vi "RVHR - New Distance.vi"(5 "Command":enum16{"Next", "Previous"}(ring), 6 "Local Data in":T3, 7 "UI Refs":T2, 8 "error in (no error)":errorcluster, 11 "Supervisory Config Cluster In":T1) -> (0 "error out":errorcluster, 3 "New Distance":dbl, 4 "Local Data out":T3)   [LabVIEW 2024]
uses:
  Controls/RVHR - Local Data.ctl
  Controls/Test Cluster.ctl
  Controls/Excluded Information.ctl
  Controls/Language.ctl
  Controls/Device_Type.ctl
  <vilib>/Utility/miscctls.llb/LVRectTypeDef.ctl
  <vilib>/Utility/miscctls.llb/LVBoundsTypeDef.ctl
  Controls/RVHR - UI Refs.ctl
  Controls/RVHR - Reporting Settings.ctl
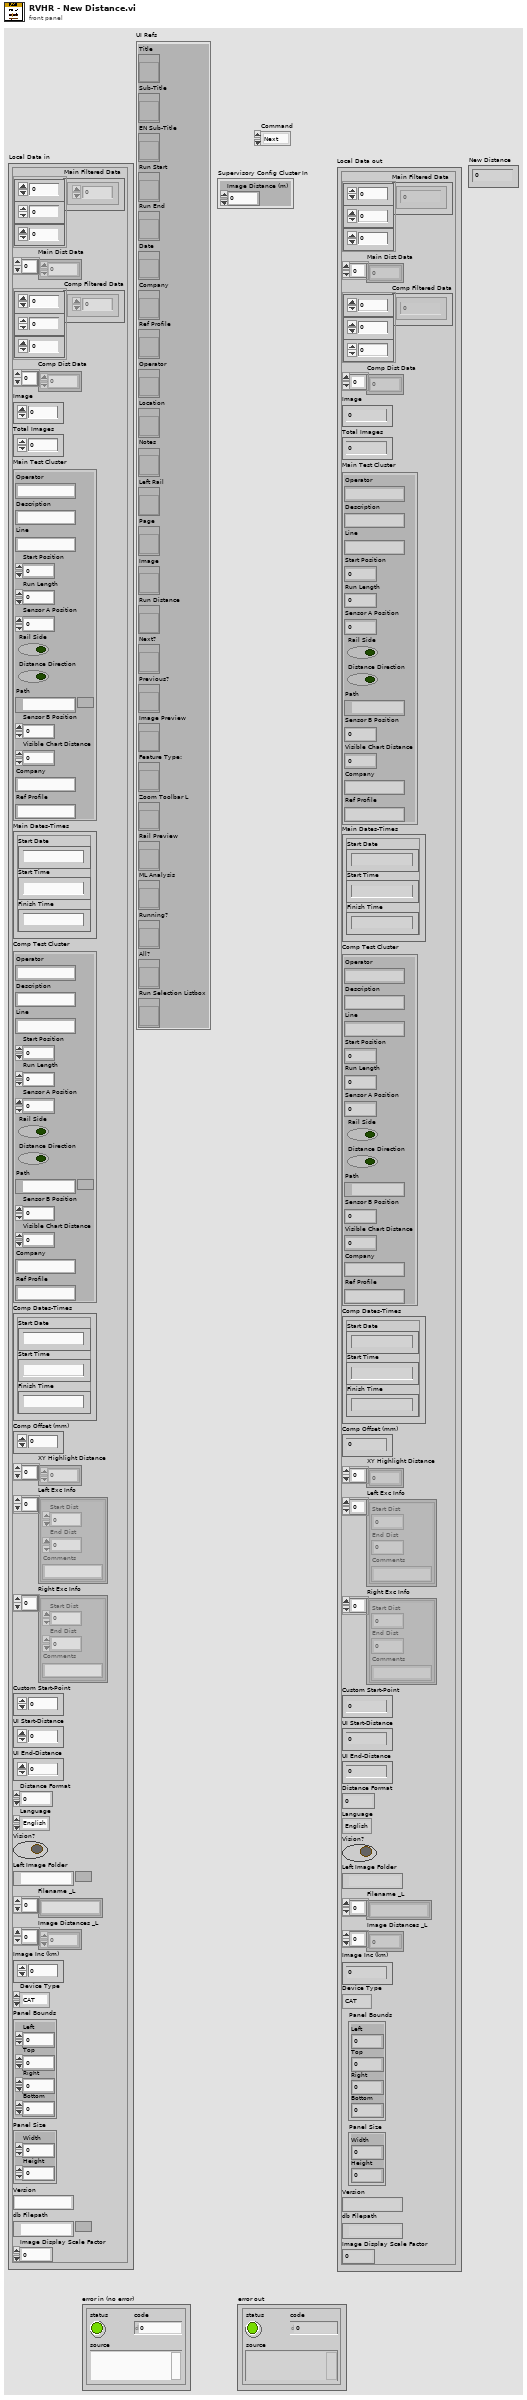
[diagram p1: front panel]
types:
  T1 = typedef "RVHR - Reporting Settings.ctl" = cluster{"Image Distance (m)":dbl}
  T2 = typedef "RVHR - UI Refs.ctl" = cluster{"Title":refnum<vi>, "Sub-Title":refnum<vi>, "EN Sub-Title":refnum<vi>, "Run Start":refnum<vi>, "Run End":refnum<vi>, "Date":refnum<vi>, "Company":refnum<vi>, "Ref Profile":refnum<vi>, "Operator":refnum<vi>, "Location":refnum<vi>, "Notes":refnum<vi>, "Left Rail":refnum<vi>, "Page":refnum<vi>, "Image":refnum<vi>, "Run Distance":refnum<vi>, "Next?":refnum<vi>, "Previous?":refnum<vi>, "Image Preview":refnum<vi>, "Feature Type:":refnum<vi>, "Zoom Toolbar L":refnum<vi>, "Rail Preview":refnum<vi>, "ML Analysis":refnum<vi>, "Running?":refnum<vi>, "All?":refnum<vi>, "Run Selection Listbox":refnum<vi>}
  T3 = typedef "RVHR - Local Data.ctl" = cluster{"Main Filtered Data":dbl[][][], "Main Dist Data":dbl[], "Comp Filtered Data":dbl[][][], "Comp Dist Data":dbl[], "Image":u16, "Total Images":u16, "Main Test Cluster":T4, "Main Dates-Times":cluster{"Start Date":string, "Start Time":string, "Finish Time":string}, "Comp Test Cluster":T4, "Comp Dates-Times":cluster{"Start Date":string, "Start Time":string, "Finish Time":string}, "Comp Offset (mm)":i64, "XY Highlight Distance":dbl[], "Left Exc Info":T5[], "Right Exc Info":T5[], "Custom Start-Point":dbl, "UI Start-Distance":dbl, "UI End-Distance":dbl, "Distance Format":u8, "Language":T6, "Vision?":bool, "Left Image Folder":path, "Filename _L":string[], "Image Distances _L":dbl[], "Image Inc (km)":dbl, "Device Type":T7, "Panel Bounds":T8, "Panel Size":T9, "Version":string, "db Filepath":path, "Image Display Scale Factor":dbl}
  T4 = typedef "Test Cluster.ctl" = cluster{"Operator":string, "Description":string, "Line":string, "Start Position":dbl, "Run Length":dbl, "Sensor A Position":dbl, "Rail Side":bool, "Distance Direction":bool, "Path":path, "Sensor B Position":dbl, "Visible Chart Distance":dbl, "Company":string, "Ref Profile":string}
  T5 = typedef "Excluded Information.ctl" = cluster{"Start Dist":dbl, "End Dist":dbl, "Comments":string}
  T6 = typedef "Language.ctl" = enum16{"English", "Chinese", "German"}
  T7 = typedef "Device_Type.ctl" = enum16{"CAT", "Bi-CAT", "YRCA", "RCA", "RV-HR", "TV-HR"}
  T8 = typedef "LVRectTypeDef.ctl" = cluster{"Left":i16, "Top":i16, "Right":i16, "Bottom":i16}
  T9 = typedef "LVBoundsTypeDef.ctl" = cluster{"Width":u32, "Height":u32}
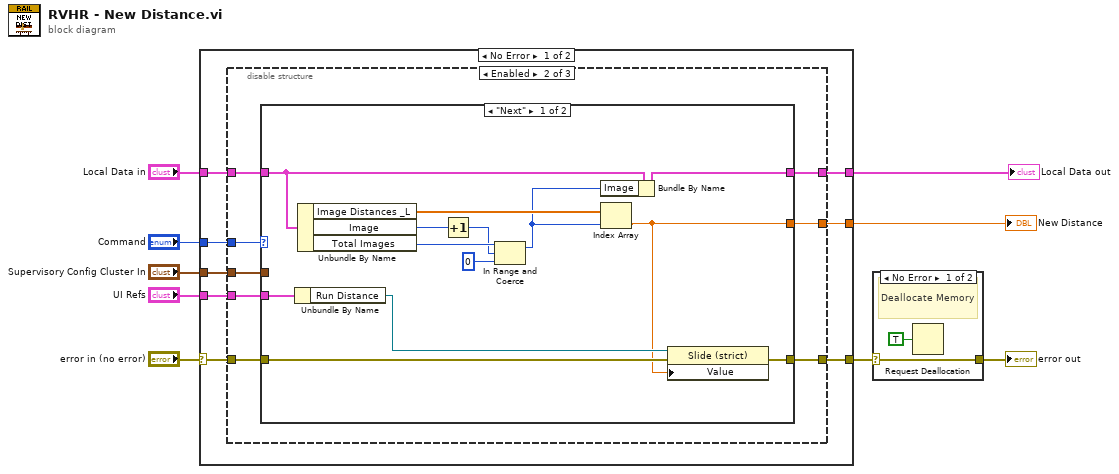
[diagram p0: block diagram]
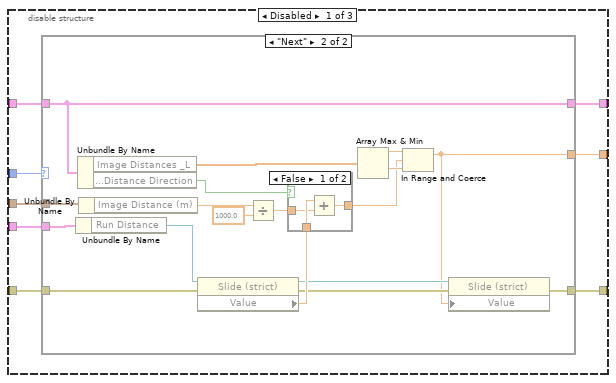
[diagram p3: hidden frame]
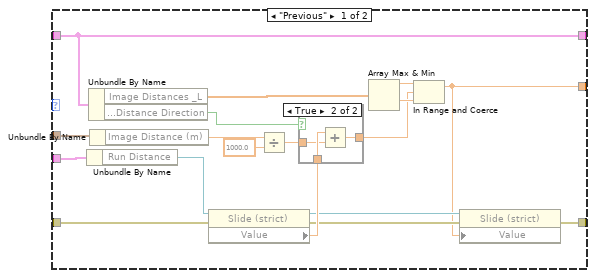
[diagram p4: hidden frame]
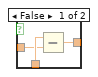
[diagram p5: hidden frame]
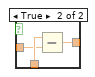
[diagram p6: hidden frame]
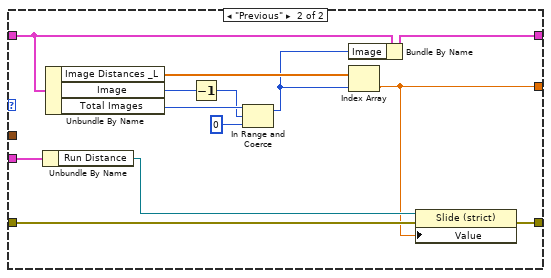
[diagram p7: hidden frame]
diagram:
  n1 = case shown="No Error" "error in (no error)" {
    selector: "error in (no error)" -> [w16 w108]
    tunnel: "UI Refs" -> [w17 _]
    tunnel: [w13 w109] -> w4
    tunnel: "Local Data in" -> [w12 w109]
    tunnel: [w15 w108] -> w2
    tunnel: [w11 _] -> w9
    tunnel: "Command" -> [w14 _]
    tunnel: "Supervisory Config Cluster In" -> [w10 _]
    frame No Error {
      n2 = disable-structure shown="Enabled" {
        disable-tunnel: w17 -> [w25 w81 _]
        disable-tunnel: w16 -> [w24 w80 _]
        disable-tunnel: [w23 w79 _] -> w15
        disable-tunnel: w14 -> [w22 w78 _]
        disable-tunnel: [w21 w77 _] -> w13
        disable-tunnel: w12 -> [w20 w76 _]
        disable-tunnel: [w19 w75 _] -> w11
        disable-tunnel: w10 -> [w18 w74 _]
        frame Disabled {
          n3 = case shown="\"Next\"" w22 {
            tunnel: w25 -> [w43 w67]
            tunnel: w24 -> [w40 w64]
            tunnel: [w30 w54] -> w23
            tunnel: [w42 w66] -> w21
            tunnel: w20 -> [w42 w66]
            tunnel: [w29 w53] -> w19
            tunnel: w18 -> [w39 w63]
            frame "Previous" {
              n4 = Unbundle By Name(w43) -> ("Run Distance"=w41:refnum<vi>)
              n5 = Unbundle By Name(w42) -> ("Image Distances _L"=w36:dbl[], "Main Test Cluster.Distance Direction"=w26:bool)
              n6 = Unbundle By Name(w39) -> ("Image Distance (m)"=w37:dbl)
              n7 = property class="Slide (strict)"(reference=w41, error in=w40) -> (reference out=w31:refnum<vi>, error out=w32:errorcluster, "Value"=w38:dbl)
              n8 = Divide(x=w37, y=1000.0) -> (x/y=w28:dbl)
              n9 = case shown="True" w26 {
                tunnel: w38 -> [w46 w49]
                tunnel: [w45 w48] -> w33
                tunnel: w28 -> [w44 w47]
                frame False {
                  n10 = Subtract(x=w46, y=w44) -> (x-y=w45:dbl)
                }
                frame True {
                  n11 = Add(x=w49, y=w47) -> (x+y=w48:dbl)
                }
              }
              n12 = Array Max & Min(array=w36) -> (max value=w35:dbl, min value=w34:dbl)  [unwired: 2 out]
              n13 = In Range and Coerce(upper limit=w35, x=w33, lower limit=w34) -> (coerced(x)=w29:dbl)  [unwired: 1 out]
              n14 = property class="Slide (strict)"(reference=w31, error in=w32, "Value"=w29) -> (error out=w30:errorcluster)  [unwired: 1 out]
            }
            frame "Next" {
              n15 = Unbundle By Name(w67) -> ("Run Distance"=w65:refnum<vi>)
              n16 = Unbundle By Name(w66) -> ("Image Distances _L"=w60:dbl[], "Main Test Cluster.Distance Direction"=w50:bool)
              n17 = Unbundle By Name(w63) -> ("Image Distance (m)"=w61:dbl)
              n18 = property class="Slide (strict)"(reference=w65, error in=w64) -> (reference out=w55:refnum<vi>, error out=w56:errorcluster, "Value"=w62:dbl)
              n19 = Divide(x=w61, y=1000.0) -> (x/y=w52:dbl)
              n20 = case shown="False" w50 {
                tunnel: w62 -> [w70 w73]
                tunnel: [w69 w72] -> w57
                tunnel: w52 -> [w68 w71]
                frame False {
                  n21 = Add(x=w70, y=w68) -> (x+y=w69:dbl)
                }
                frame True {
                  n22 = Subtract(x=w73, y=w71) -> (x-y=w72:dbl)
                }
              }
              n23 = Array Max & Min(array=w60) -> (max value=w59:dbl, min value=w58:dbl)  [unwired: 2 out]
              n24 = In Range and Coerce(upper limit=w59, x=w57, lower limit=w58) -> (coerced(x)=w53:dbl)  [unwired: 1 out]
              n25 = property class="Slide (strict)"(reference=w55, error in=w56, "Value"=w53) -> (error out=w54:errorcluster)  [unwired: 1 out]
            }
          }
        }
        frame Enabled {
          n26 = case shown="\"Next\"" w78 {
            tunnel: w81 -> [w94 w107]
            tunnel: w80 -> [w91 w104]
            tunnel: [w90 w103] -> w79
            tunnel: [w86 w99] -> w77
            tunnel: w76 -> [w93 w106]
            tunnel: [w87 w100] -> w75
            tunnel: w74 -> [_ _]
            frame "Next" {
              n27 = Unbundle By Name(w94) -> ("Run Distance"=w92:refnum<vi>)
              n28 = Unbundle By Name(w93) -> ("Image Distances _L"=w89:dbl[], "Image"=w88:u16, "Total Images"=w85:u16)
              n29 = Increment(x=w88) -> (x+1=w84:u16)
              n30 = In Range and Coerce(upper limit=w85, x=w84, lower limit=u8 0 ("x")) -> (coerced(x)=w83:u16)  [unwired: 1 out]
              n31 = Bundle By Name(cluster=w93, "Image"=w83) -> (w86:T3)
              n32 = Index Array(array=w89, index=w83) -> (element=w87:dbl)
              n33 = property class="Slide (strict)"(reference=w92, error in=w91, "Value"=w87) -> (error out=w90:errorcluster)  [unwired: 1 out]
            }
            frame "Previous" {
              n34 = Unbundle By Name(w107) -> ("Run Distance"=w105:refnum<vi>)
              n35 = Unbundle By Name(w106) -> ("Image Distances _L"=w102:dbl[], "Image"=w101:u16, "Total Images"=w98:u16)
              n36 = Decrement(x=w101) -> (x-1=w97:u16)
              n37 = In Range and Coerce(upper limit=w98, x=w97, lower limit=u8 0 ("x")) -> (coerced(x)=w96:u16)  [unwired: 1 out]
              n38 = Bundle By Name(cluster=w106, "Image"=w96) -> (w99:T3)
              n39 = Index Array(array=w102, index=w96) -> (element=w100:dbl)
              n40 = property class="Slide (strict)"(reference=w105, error in=w104, "Value"=w100) -> (error out=w103:errorcluster)  [unwired: 1 out]
            }
          }
        }
        frame Disabled {
        }
      }
    }
    frame Error {
    }
  }
  "New Distance" <- w9
  "Local Data out" <- w4
  n41 = case shown="No Error" w2 {
    selector: w2 -> [w110 w112]
    tunnel: [w110 w112] -> w1
    frame No Error {
      # "Deallocate Memory"
      n42 = Request Deallocation(TRUE ("flag")) -> ()
    }
    frame Error {
    }
  }
  "error out" <- w1
